vi "Level Meter Device (Set).vi"(6 "ISOBUS address":T10=-1 caption="ISOBUS address (-1)", 8 "error in":errorcluster, 10 "Level Meter":T3, 11 "Mercury Reference In":T11) -> (0 "error out":errorcluster, 2 "Response":T1, 3 "Mercury Reference Out":T11, 4 "Valid?":T2)   [LabVIEW 2013, in "Mercury iXX.lvlib" / "Level Meter.lvlib"]
doc: "Set the level meter device configuration."
uses:
  <instrlib>/Mercury iXX/Public/Libraries/Level Meter.lvlib
  <instrlib>/Mercury iXX/Public/Controls/Mercury Reference.ctl
  <instrlib>/Mercury iXX/Public/Controls/Comms Transport Layer.ctl
  <instrlib>/Mercury iXX/Private/Controls/Query Dynamic Reference.ctl
  <instrlib>/Mercury iXX/Public/Controls/ISOBus Address.ctl
  <instrlib>/Mercury iXX/Public/Libraries/Level Meter/Controls/Level Meter (Set).ctl
  <instrlib>/Mercury iXX/Public/Libraries/Level Meter/Controls/Helium Configuration.ctl
  <instrlib>/Mercury iXX/Public/Libraries/Level Meter/Controls/Resistance Configuration.ctl
  <instrlib>/Mercury iXX/Public/Libraries/Level Meter/Controls/Pre-Pulse.ctl
  <instrlib>/Mercury iXX/Public/Libraries/Level Meter/Controls/Pulse.ctl
  <instrlib>/Mercury iXX/Public/Libraries/Level Meter/Controls/Nitrogen Configuration.ctl
  <instrlib>/Mercury iXX/Public/Libraries/Level Meter/Controls/Frequency Configuration.ctl
  <instrlib>/Mercury iXX/Public/Controls/Is Valid LED.ctl
  <instrlib>/Mercury iXX/Public/Controls/Response String.ctl
  <instrlib>/Mercury iXX/Private/Controls/Command Verbs.ctl
  <instrlib>/Mercury iXX/Mercury iXX.lvlib
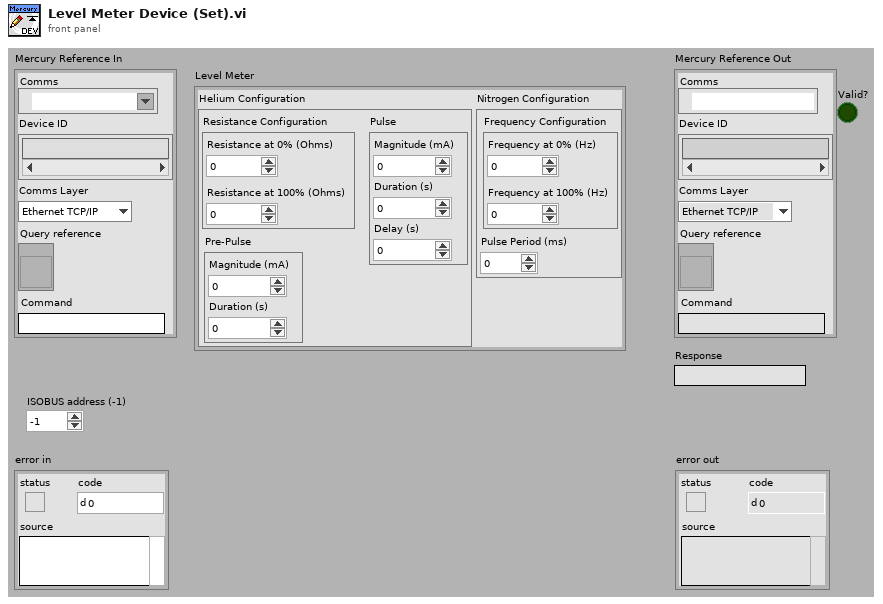
[diagram p1: front panel]
types:
  T1 = typedef "Mercury iXX.lvlib/Response String.ctl" = string
  T2 = typedef "Mercury iXX.lvlib/Is Valid LED.ctl" = bool
  T3 = typedef "Mercury iXX.lvlib/Level Meter.lvlib/Level Meter (Set).ctl" = cluster{"Helium Configuration":T4, "Nitrogen Configuration":T8}
  T4 = typedef "Mercury iXX.lvlib/Level Meter.lvlib/Helium Configuration.ctl" = cluster{"Resistance Configuration":T5, "Pre-Pulse":T6, "Pulse":T7}
  T5 = typedef "Mercury iXX.lvlib/Level Meter.lvlib/Resistance Configuration.ctl" = cluster{"Res 0%":dbl, "Res 100%":dbl}
  T6 = typedef "Mercury iXX.lvlib/Level Meter.lvlib/Pre-Pulse.ctl" = cluster{"Magnitude":dbl, "Duration":dbl}
  T7 = typedef "Mercury iXX.lvlib/Level Meter.lvlib/Pulse.ctl" = cluster{"Magnitude":dbl, "Duration":dbl, "Delay":dbl}
  T8 = typedef "Mercury iXX.lvlib/Level Meter.lvlib/Nitrogen Configuration.ctl" = cluster{"Frequency Configuration":T9, "Pulse Period":dbl}
  T9 = typedef "Mercury iXX.lvlib/Level Meter.lvlib/Frequency Configuration.ctl" = cluster{"Freq 0%":dbl, "Freq 100%":dbl}
  T10 = typedef "Mercury iXX.lvlib/ISOBus Address.ctl" = i32
  T11 = typedef "Mercury iXX.lvlib/Mercury Reference.ctl" = cluster{"Comms":refnum<visa-resource-name>, "Device ID":string[], "Comms Layer":T12, "Command":string, "Query reference":T13}
  T12 = typedef "Mercury iXX.lvlib/Comms Transport Layer.ctl" = enum16{"Ethernet TCP/IP", "USB", "ISOBus - RS-232", "GPIB"}
  T13 = typedef "Mercury iXX.lvlib/Query Dynamic Reference.ctl" = refnum<vi>
  T14 = typedef "Mercury iXX.lvlib/Command Verbs.ctl" = string
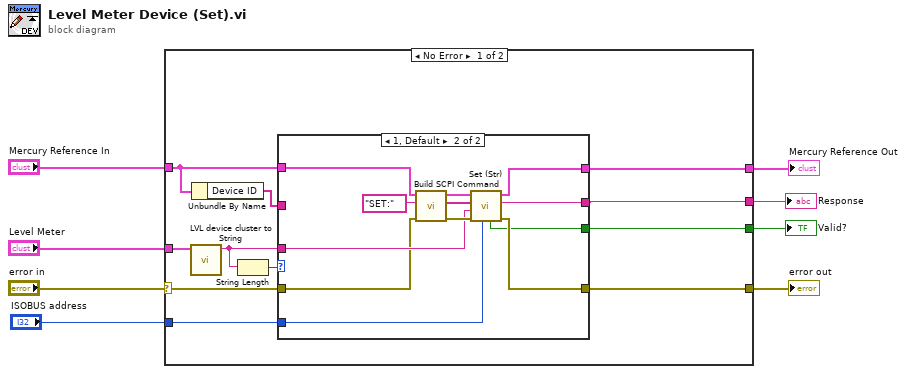
[diagram p0: block diagram]
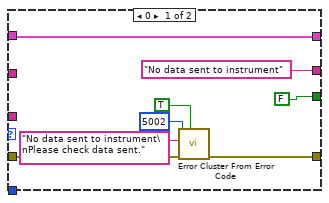
[diagram p2: hidden frame]
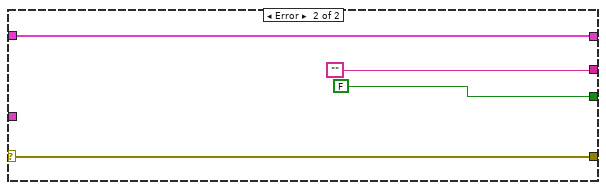
[diagram p3: hidden frame]
diagram:
  n1 = case shown="No Error" "error in" {
    selector: "error in" -> [w19 w42]
    tunnel: "Mercury Reference In" -> [w14 w43]
    tunnel: [w15 w43] -> w7
    tunnel: [w16 w42] -> w6
    tunnel: "ISOBUS address" -> [w18 _]
    tunnel: [w9 ""] -> w2
    tunnel: [w10 FALSE ("Valid?")] -> w3
    tunnel: "Level Meter" -> [w11 _]
    frame No Error {
      n2 = call <instrlib>:"LVL device cluster to String.vi"("Level Meter"=w11) -> ("Data to send"=w12:string)  [unwired: 1 in, 9 out]
      n3 = Unbundle By Name(w14) -> ("Device ID"=w17:string[])
      n4 = String Length(string=w12) -> (length=w13:i32)
      n5 = case shown="1, Default" w13 {
        tunnel: ["No data sent to instrument" ("Data") w29] -> w9
        tunnel: w14 -> [w27 w35]
        tunnel: w17 -> [_ _]
        tunnel: w18 -> [_ w31]
        tunnel: w19 -> [w25 w33]
        tunnel: [w26 w32] -> w16
        tunnel: [w27 w28] -> w15
        tunnel: w12 -> [_ w34]
        tunnel: [FALSE ("Valid?") w30] -> w10
        frame 0 {
          n6 = call <vilib>:"Error Cluster From Error Code.vi"("show call chain? (False)"=TRUE, "error in (no error)"=w25, "error message (\"\")"="No data sent to instrument\nPlease check data sent." ("error message (\"\")"), "error code (0)"=5002) -> ("error out"=w26:errorcluster)  [unwired: 5 out]
        }
        frame 1, Default {
          n7 = call <instrlib>:"Build SCPI Command.vi"("error in"=w33, "Verb"=T14 "SET:", "Mercury Reference In"=w35) -> ("error out"=w37:errorcluster, "SCPI Message(s)"=w38:string[], "Mercury Reference Out"=w39:T11)  [unwired: 1 in, 5 out]
          n8 = call <instrlib>:"Set (Str).vi"("ISOBUS address"=w31, "error in"=w37, "Command Value (Str)"=w34, "SCPI Message(s)"=w38, "Mercury Reference In"=w39) -> ("error out"=w32:errorcluster, "Response"=w29:T1, "Mercury Reference Out"=w28:T11, "Valid?"=w30:T2)  [unwired: 3 out]
        }
      }
    }
    frame Error {
    }
  }
  "Mercury Reference Out" <- w7
  "error out" <- w6
  "Valid?" <- w3
  "Response" <- w2
